vi "LibXML_OpenXMLFile.vi"(8 "error in":errorcluster, 11 "file path":path) -> (0 "error out":errorcluster, 2 "new file path":path=path "D:/bhs/programming/XML-toolkit/personnel.xml", 3 "doc":u32)   [LabVIEW 2019, in "Tools.lvlib" / "LibXML.lvlib"]
doc: "Loads the XML-file into memory.\nWhen using \"Assign schema\" the Schema-Cluster should be filled in, the schema referred to inside the xml file will be overruled. This way one can be sure that the right (your) xsd is used for validation.\nSchemalocation should hold the exact schemalocation; The namespac- uri should be the same as used in the xml-file. Prefix is not used here."
uses:
  LibXML.lvlib
  <vilib>/Utility/error.llb/Trim Whitespace.vi
  Tools.lvlib
  dll/libxml2.dll
panel:
  # "This software is FREE licensed under the GNU Lesser General Public License (see license.txt)."
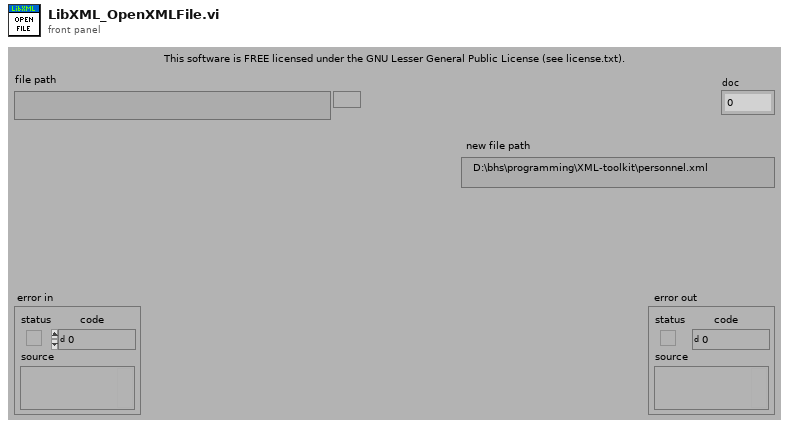
[diagram p1: front panel]
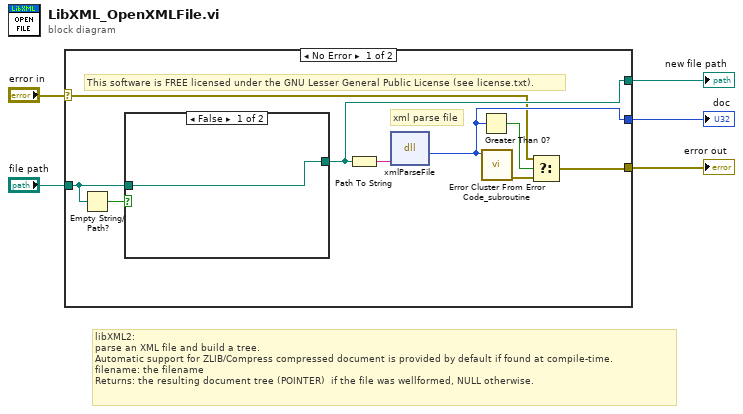
[diagram p0: block diagram]
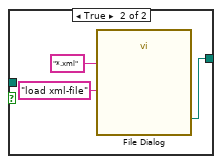
[diagram p2: hidden frame]
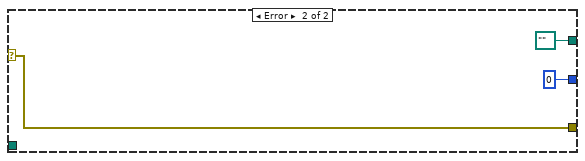
[diagram p3: hidden frame]
diagram:
  # "libXML2:\nparse an XML file and build a tree. \nAutomatic support for ZLIB/Compress compressed document is provided by default if found at compile-time.\nfilename:\tthe filename\nReturns:\tthe resulting document tree (POINTER)  if the file was wellformed, NULL otherwise."
  n1 = case shown="No Error" "error in" {
    selector: "error in" -> [w6 w21]
    tunnel: [w10 w21] -> w5
    tunnel: [w9 u32 0] -> w3
    tunnel: "file path" -> [w8 _]
    tunnel: [w7 path "" ("file path (dialog if empty)")] -> w1
    frame No Error {
      # "xml parse file"
      # "This software is FREE licensed under the GNU Lesser General Public License (see license.txt)."
      n2 = Empty String/Path?(string/path=w8) -> (empty?=w14:bool)
      n3 = case shown="False" w14 {
        tunnel: w8 -> [w15 _]
        tunnel: [w15 w18] -> w7
        frame False {
        }
        frame True {
          n4 = call "File Dialog"("prompt"="load xml-file", "pattern (all files)"="*.xml" ("pattern")) -> ("selected path"=w18:path)  [unwired: 10 in, 3 out]
        }
      }
      n5 = Path To String(path=w7) -> (string=w11:string)
      n6 = dll-call lib="C:/Projects/_Prywatne/MyCIT/Framework/Tools/XML/LibXML/dll/libxml2.dll" fn="xmlParseFile"("filename"=w11) -> ("return type"=w9:u32)  [unwired: 4 in, 2 out]
      n7 = Greater Than 0?(x=w9) -> (x > 0?=w13:bool)
      n8 = call "Error Cluster From Error Code_subroutine.vi"("error code (0)"=w9) -> ("error out"=w12:errorcluster)  [unwired: 8 in]
      n9 = Select(t=w6, s=w13, f=w12) -> (s? t:f=w10:errorcluster)
    }
    frame Error {
    }
  }
  "error out" <- w5
  "doc" <- w3
  "new file path" <- w1
